vi "RetaBola.vi"(4 "DistInFrontGoal":dbl=90.0 format="%#_13g", 5 "Meio?":bool=TRUE, 6 "Goal Width":u32, 7 "Field Lenght":u32, 8 "Vy bola":dbl format="%#_13g", 9 "Vx bola":dbl format="%#_13g", 10 "Y bola":dbl format="%#_13g", 11 "X bola":dbl format="%#_13g") -> (0 "Orientação":dbl format="%#_13g", 1 "Low ball velocity?":bool, 2 "Y goleiro":dbl format="%#_13g", 3 "X goleiro":dbl format="%#_13g")   [LabVIEW 2023]
uses:
  Utilities_class/Utilities.lvclass
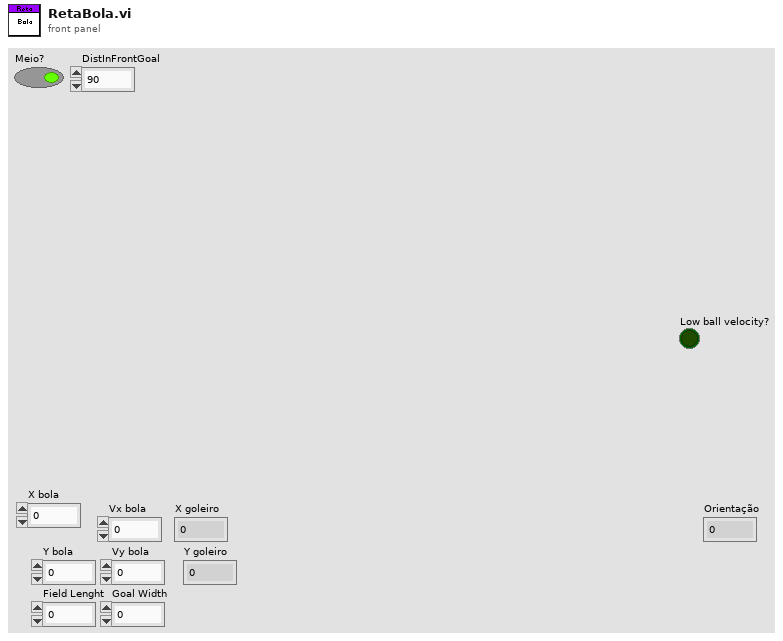
[diagram p1: front panel]
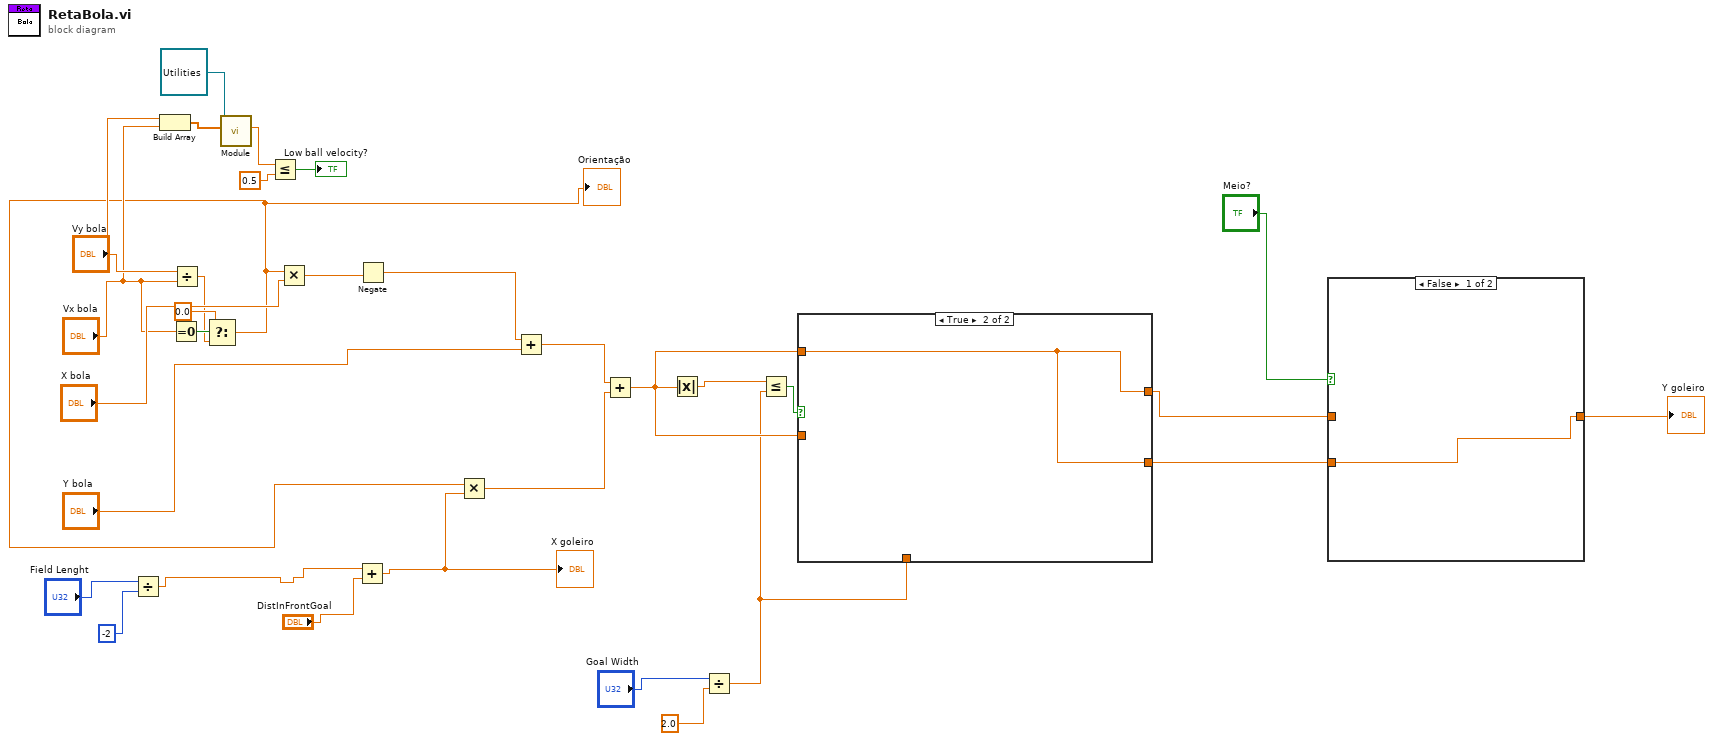
[diagram p0: block diagram]
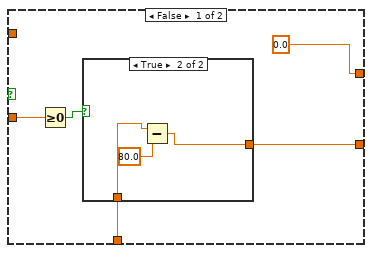
[diagram p3: hidden frame]
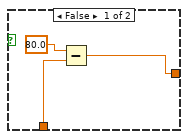
[diagram p4: hidden frame]
diagram:
  n1 = Divide(x="Field Lenght", y=-2 ("Numeric")) -> (x/y=w19:dbl)
  n2 = Build Array("Vy bola", "Vx bola") -> (w7:dbl[])
  n3 = Equal To 0?(x="Vx bola") -> (x = 0?=w12:bool)
  n4 = Divide(x="Vy bola", y="Vx bola") -> (x/y=w10:dbl)
  n5 = Select(t=0.0, s=w12, f=w10) -> (s? t:f=w3:dbl)
  "Orientação" <- w3
  n6 = call-dynamic "Module.vi"("2D vector"=w7, "Utilities in"=refnum<class "Utilities.lvclass"> refnum) -> ("Modulo"=w6:dbl)  [unwired: 7 in, 2 out]
  n7 = Less Or Equal?(x=w6, y=0.5) -> (x <= y?=→"Low ball velocity?":bool)
  n8 = Multiply(x=w3, y="X bola") -> (x*y=w30:dbl)
  n9 = Add(x=w19, y="DistInFrontGoal") -> (x+y=w26:dbl)
  "X goleiro" <- w26
  n10 = Negate(x=w30) -> (-x=w29:dbl)
  n11 = Multiply(x=w3, y=w26) -> (x*y=w24:dbl)
  n12 = Add(x=w29, y="Y bola") -> (x+y=w25:dbl)
  n13 = Add(x=w25, y=w24) -> (x+y=w15:dbl)
  n14 = Absolute Value(x=w15) -> (abs(x)=w21:dbl)
  n15 = Divide(x="Goal Width", y=2.0) -> (x/y=w14:dbl)
  n16 = Less Or Equal?(x=w21, y=w14) -> (x <= y?=w20:bool)
  n17 = case shown="True" w20 {
    tunnel: [0.0 w44] -> w17
    tunnel: w15 -> [_ w44]
    tunnel: w15 -> [w36 _]
    tunnel: w14 -> [w34 _]
    tunnel: [w33 w44] -> w13
    frame False {
      n18 = Greater Or Equal To 0?(x=w36) -> (x >= 0?=w35:bool)
      n19 = case shown="True" w35 {
        tunnel: w34 -> [w39 w43]
        tunnel: [w38 w41] -> w33
        frame False {
          n20 = Subtract(x=80.0 ("y"), y=w39) -> (x-y=w38:dbl)
        }
        frame True {
          n21 = Subtract(x=w43, y=80.0 ("x-y")) -> (x-y=w41:dbl)
        }
      }
    }
    frame True {
    }
  }
  n22 = case shown="False" "Meio?" {
    tunnel: w17 -> [_ w46]
    tunnel: [w45 w46] -> w16
    tunnel: w13 -> [w45 _]
    frame False {
    }
    frame True {
    }
  }
  "Y goleiro" <- w16
